vi "Format Container Into String.vi"(0 "initial string":string, 2 "format string":string, 7 "error in":errorcluster, 11 "input":variant) -> (4 "resulting string":string, 8 "error out":errorcluster)   [LabVIEW 2015, in "LV String Utils v1.lvlib"]
doc: "Converts anything to string according the formating string. String representation is as much compatible with Python repr as possible."
uses:
  LV String Utils v1.lvlib
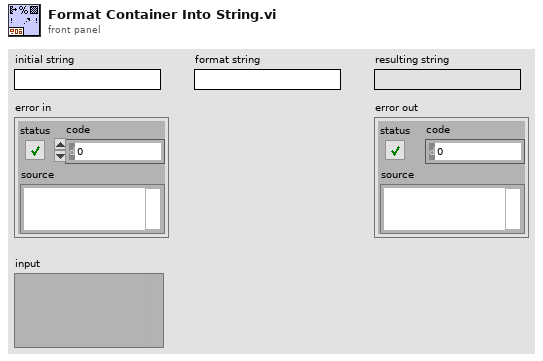
[diagram p1: front panel]
types:
  T1 = typedef "Type Descriptor Header__ogtk.ctl" = cluster{"length":u16, "private":u8, "type":T2, "# elements":u16}
  T2 = typedef "Type Descriptor Enumeration__ogtk.ctl" = enum8{"<Null>", "I8", "I16", "I32", "I64", "U8", "U16", "U32", "U64", "SGL", "DBL", "EXT", "CSG", "CDB", "CXT", "0x0F", "0x10", "0x11", "0x12", "0x13", "0x14", "Enum U8", "Enum U16", "Enum U32", "Enum U64", "SGL PQ", "DBL PQ", "EXT PQ", "CSG PQ", "CDB PQ", "CXT PQ", "0x1F", "0x20", "Boolean", "0x22", "0x23", "0x24", "0x25", "0x26", "0x27", "0x28", "0x29", "0x2A", "0x2B", "0x2C", "0x2D", "0x2E", "0x2F", "String", "0x31", "Path", "Pict", "0x34", "0x35", "0x36", "DAQ", "0x38", "0x39", "0x3A", "0x3B", "0x3C", "0x3D", "0x3E", "0x3F", "Array", "0x41", "0x42", "0x43", "0x44", "0x45", "0x46", "0x47", "0x48", "0x49", "0x4A", "0x4B", "0x4C", "0x4D", "0x4E", "0x4F", "Cluster", "0x51", "0x52", "Variant", "Waveform", "0x55", "0x56", "0x57", "0x58", "0x59", "0x5A", "0x5B", "0x5C", "0x5D", "0x5E", "0x5F", "0x60", "0x61", "0x62", "0x63", "0x64", "0x65", "0x66", "0x67", "0x68", "0x69", "0x6A", "0x6B", "0x6C", "0x6D", "0x6E", "0x6F", "Refnum"}
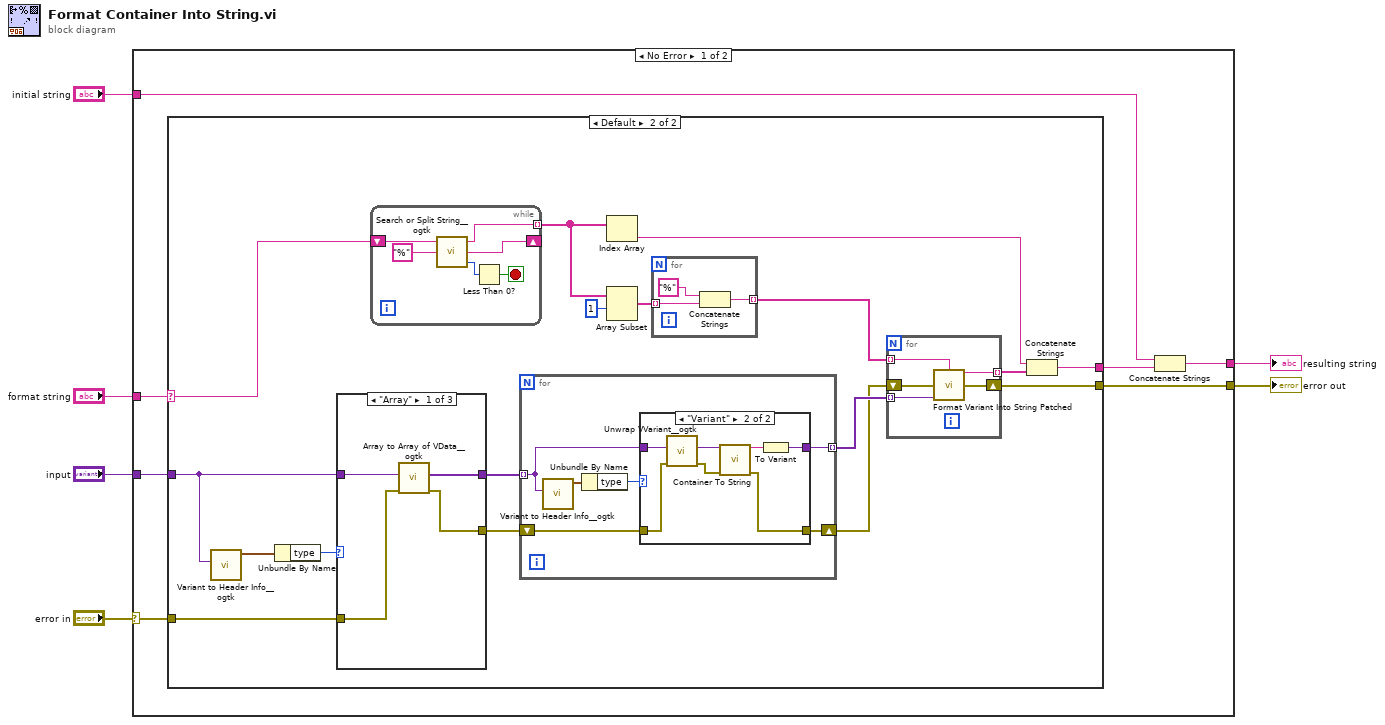
[diagram p0: block diagram]
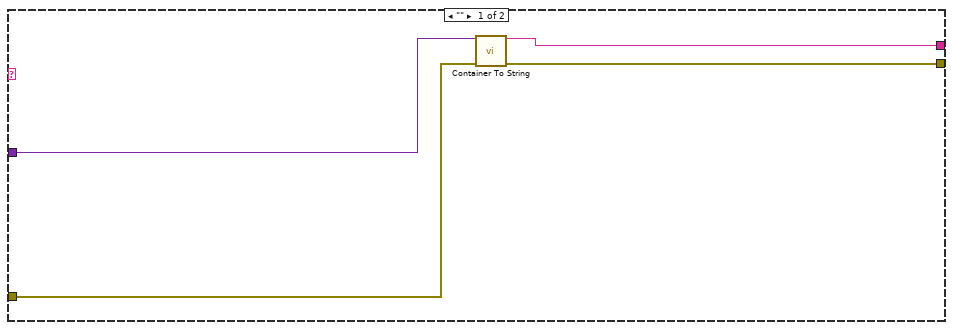
[diagram p2: hidden frame]
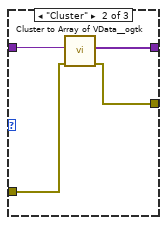
[diagram p4: hidden frame]
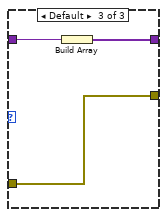
[diagram p5: hidden frame]
diagram:
  n1 = case shown="No Error" "error in" {
    selector: "error in" -> [w10 w75]
    tunnel: "input" -> [w13 _]
    tunnel: [w12 w75] -> w5
    tunnel: "format string" -> [w11 _]
    tunnel: [w8 _] -> w3
    tunnel: "initial string" -> [w7 _]
    frame No Error {
      n2 = case shown="Default" w11 {
        selector: w11 -> [_ w18]
        tunnel: w13 -> [w17 w27]
        tunnel: [w14 w21] -> w12
        tunnel: w10 -> [w15 w20]
        tunnel: [w16 w19] -> w9
        frame "" {
          n3 = call "Container To String.vi"("variant"=w17, "error in (no error)"=w15) -> ("string"=w16:string, "error out"=w14:errorcluster)  [unwired: 11 in, 1 out]
        }
        frame Default {
          n4 = call <userlib>:"Variant to Header Info__ogtk.vi"("Variant"=w27) -> ("Type Descriptor Header"=w28:T1)  [unwired: 3 in, 2 out]
          n5 = Unbundle By Name(w28) -> ("type"=w26:T2)
          n6 = case shown="\"Array\"" w26 {
            tunnel: w27 -> [w53 w57 w60]
            tunnel: [w52 w56 w59] -> w25
            tunnel: [w51 w54 w58] -> w23
            tunnel: w20 -> [w50 w55 w58]
            frame "Array" {
              n7 = call <userlib>:"Array to Array of VData__ogtk.vi"("error in (no error)"=w50, "MultiD Array"=w53) -> ("error out"=w51:errorcluster, "1D Array of Variants"=w52:variant[])  [unwired: 8 in]
            }
            frame "Cluster" {
              n8 = call <userlib>:"Cluster to Array of VData__ogtk.vi"("error in (no error)"=w55, "Cluster"=w57) -> ("error out"=w54:errorcluster, "Array of VData"=w56:variant[])  [unwired: 8 in]
            }
            frame Default {
              n9 = Build Array(w60) -> (w59:variant[])
            }
          }
          n10 = while {
            shift-right: [w70] -> _
            shift-left: w18 -> [w73]
            tunnel: [w69] -> w32 mode=indexing
            stop <- w74 stop-if-true
            n11 = call <userlib>:"Search or Split String__ogtk.vi"("search string/char (-)"="%", "string"=w73) -> ("offset after match"=w71:i32, "substring after match"=w70:string, "substring before match"=w69:string)  [unwired: 1 in]
            n12 = Less Than 0?(x=w71) -> (x < 0?=w74:bool)
          }
          n13 = for {
            tunnel: w25 -> [w37] mode=indexing
            tunnel: [w38] -> w24 mode=indexing
            shift-right: [w35] -> w22
            shift-left: w23 -> [w36]
            n14 = call <userlib>:"Variant to Header Info__ogtk.vi"("Variant"=w37) -> ("Type Descriptor Header"=w40:T1)  [unwired: 3 in, 2 out]
            n15 = Unbundle By Name(w40) -> ("type"=w39:T2)
            n16 = case shown="\"Variant\"" w39 {
              tunnel: [w42 w43] -> w38
              tunnel: w37 -> [w42 w47]
              tunnel: w36 -> [w41 w46]
              tunnel: [w41 w45] -> w35
              frame Default {
              }
              frame "Variant" {
                n17 = call <userlib>:"Unwrap VVariant__ogtk.vi"("error in (no error)"=w46, "VVariant"=w47) -> ("error out"=w49:errorcluster, "Variant"=w48:variant)  [unwired: 8 in]
                n18 = call "Container To String.vi"("variant"=w48, "error in (no error)"=w49) -> ("string"=w44:string, "error out"=w45:errorcluster)  [unwired: 11 in, 1 out]
                n19 = To Variant(anything=w44) -> (Variant=w43:variant)
              }
            }
          }
          n20 = Index Array(array=w32) -> (element=w29:string)  [unwired: 1 in]
          n21 = Array Subset(array=w32, index=1) -> (w33:string[])  [unwired: 1 in]
          n22 = for {
            tunnel: w33 -> [w68] mode=indexing
            tunnel: [w66] -> w31 mode=indexing
            n23 = Concatenate Strings("%" ("search string/char (-)"), w68) -> (w66:string)
          }
          n24 = for {
            tunnel: w31 -> [w62] mode=indexing
            tunnel: w24 -> [w65] mode=indexing
            shift-right: [w63] -> w21
            shift-left: w22 -> [w64]
            tunnel: [w61] -> w30 mode=indexing
            n25 = call "Format Variant Into String Patched.vi"("Format String"=w62, "error in (no error)"=w64, "Variant"=w65) -> ("Output String"=w61:string, "error out"=w63:errorcluster)  [unwired: 11 in]
          }
          n26 = Concatenate Strings(w29, w30) -> (w19:string)
        }
      }
      n27 = Concatenate Strings(w7, w9) -> (w8:string)
    }
    frame Error {
    }
  }
  "resulting string" <- w3
  "error out" <- w5
